vi "metrics.vi"(9 "Бит неч":dbl, 10 "Бит чет":dbl) -> (2 "Возможные\nметрики ребер":dbl[](array[numeric]))   [LabVIEW 2017]
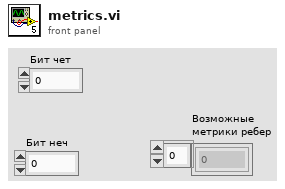
[diagram p1: front panel]
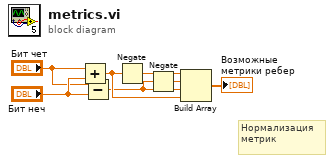
[diagram p0: block diagram]
diagram:
  # "Нормализация\nметрик"
  n1 = Add(x="Бит чет", y="Бит неч") -> (x+y=w6:dbl)
  n2 = Subtract(x="Бит чет", y="Бит неч") -> (x-y=w4:dbl)
  n3 = Negate(x=w6) -> (-x=w7:dbl)
  n4 = Negate(x=w4) -> (-x=w5:dbl)
  n5 = Build Array(w7, w5, w4, w6) -> (→"Возможные\nметрики ребер":dbl[])
